vi "path to string array.vi"() -> ()   [LabVIEW 2010, in "util.lvlib"]
uses:
  util.lvlib
panel:
  in  "path":path
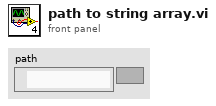
[diagram p1: front panel]
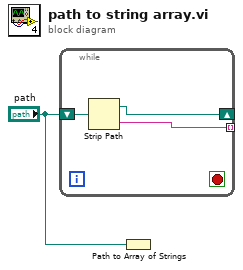
[diagram p0: block diagram]
diagram:
  n1 = while {
    shift-right: [w3] -> _
    shift-left: "path" -> [w4]
    tunnel: [w2] -> _ mode=indexing
    stop <- _ stop-if-true
    n2 = Strip Path(path=w4) -> (stripped path=w3:path, name=w2:string)
  }
  n3 = Path to Array of Strings(0:"path") -> ()  [unwired: 2 out]
